vi "灵敏度判定.vi"(0 "曲线引用":refnum<vi>, 1 "灵敏度":T1, 3 "错误输入":errorcluster) -> (7 "曲线引用输出":refnum<vi>, 8 "OK？":bool, 10 "错误输出":errorcluster)   [LabVIEW 2018]
uses:
  Global_Variable/Global.vi
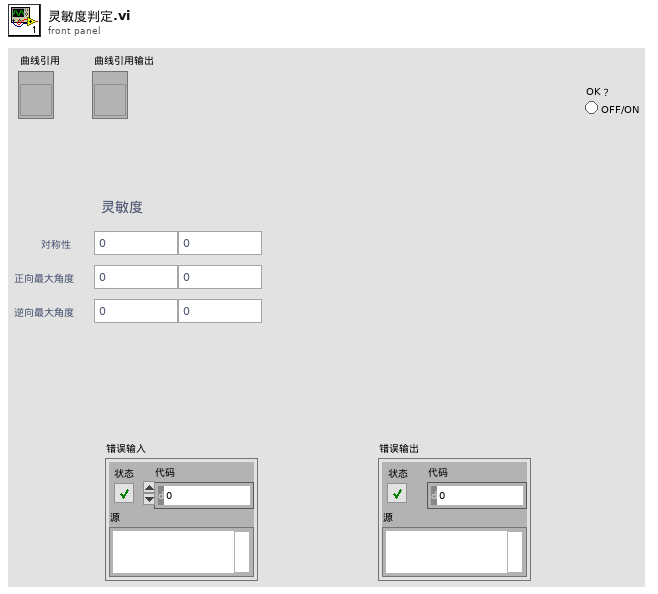
[diagram p1: front panel]
types:
  T1 = cluster{"         对称性":cluster{"下限":dbl, "上限":dbl}, "正向最大角度":cluster{"下限":dbl, "上限":dbl}, "逆向最大角度":cluster{"下限":dbl, "上限":dbl}}
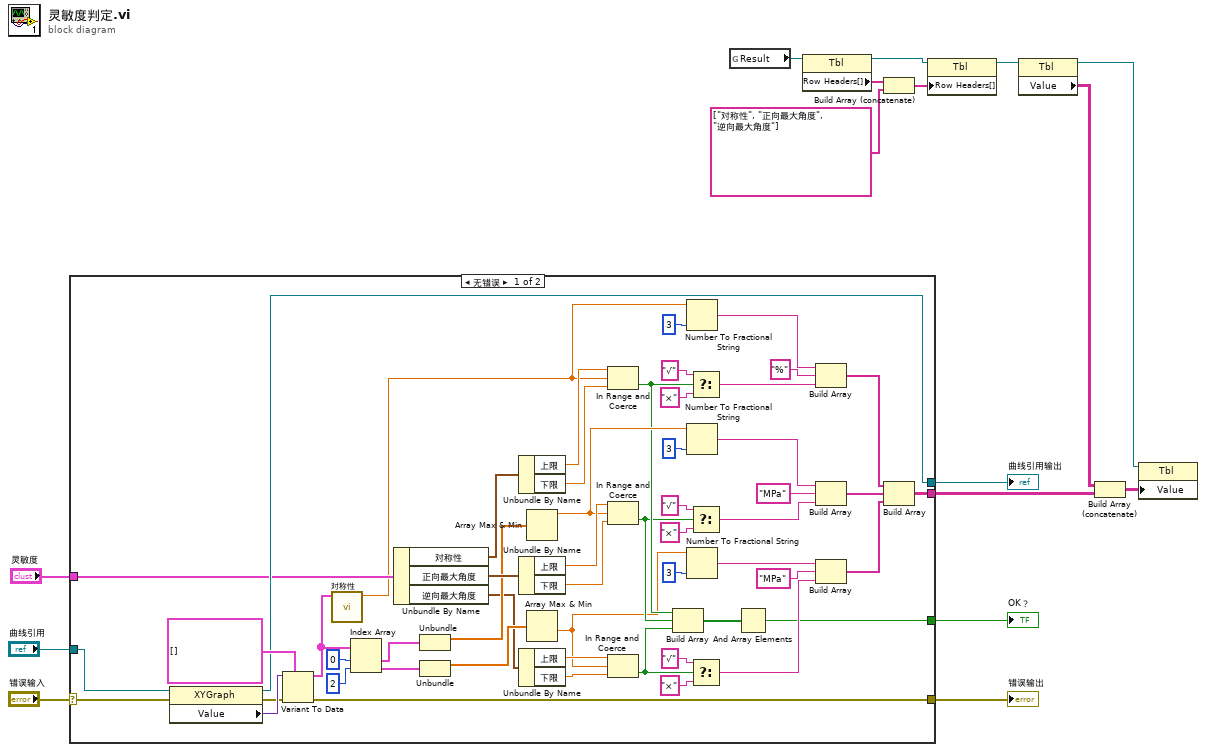
[diagram p0: block diagram]
diagram:
  n1 = case shown="无错误" "错误输入" {
    selector: "错误输入" -> [w68 w72]
    tunnel: [w65 w72] -> w15
    tunnel: "曲线引用" -> [w64 w71]
    tunnel: [w67 w71] -> w13
    tunnel: [w19 _] -> w12
    tunnel: "灵敏度" -> [w63 _]
    tunnel: [w18 _] -> w8
    frame No Error {
      n2 = property class="XYGraph"(reference=w64, error in=w68) -> (reference out=w67:refnum<vi>, error out=w66:errorcluster, "Value"=w70:variant)
      n3 = Variant To Data(error in=w66, type=cluster{dbl[], dbl[]}[] [], Variant=w70) -> (data=w52:cluster{dbl[], dbl[]}[], error out=w65:errorcluster)
      n4 = call "对称性.vi"("XY图"=w52) -> ("对称性"=w59:dbl)  [unwired: 8 in, 2 out]
      n5 = Index Array(array=w52, index #1=0 ("索引"), index #2=2 ("索引")) -> (element #1=w28:cluster{dbl[], dbl[]}, element #2=w27:cluster{dbl[], dbl[]})
      n6 = Unbundle By Name(w63) -> ("对称性"=w62:cluster{"下限":dbl, "上限":dbl}, "正向最大角度"=w43:cluster{"下限":dbl, "上限":dbl}, "逆向最大角度"=w31:cluster{"下限":dbl, "上限":dbl})
      n7 = Unbundle(w28) -> (w42:dbl[])  [unwired: 1 out]
      n8 = Unbundle(w27) -> (w32:dbl[])  [unwired: 1 out]
      n9 = Unbundle By Name(w62) -> ("上限"=w61:dbl, "下限"=w60:dbl)
      n10 = Unbundle By Name(w43) -> ("上限"=w44:dbl, "下限"=w45:dbl)
      n11 = Unbundle By Name(w31) -> ("上限"=w40:dbl, "下限"=w39:dbl)
      n12 = Array Max & Min(array=w42) -> (max value=w41:dbl)  [unwired: 3 out]
      n13 = Array Max & Min(array=w32) -> (min value=w17:dbl)  [unwired: 3 out]
      n14 = In Range and Coerce(upper limit=w61, x=w59, lower limit=w60) -> (In Range?=w25:bool)  [unwired: 1 out]
      n15 = In Range and Coerce(upper limit=w44, x=w41, lower limit=w45) -> (In Range?=w23:bool)  [unwired: 1 out]
      n16 = In Range and Coerce(upper limit=w40, x=w17, lower limit=w39) -> (In Range?=w21:bool)  [unwired: 1 out]
      n17 = Build Array(w25, w23, w21) -> (w20:bool[])
      n18 = Number To Fractional String(number=w59, precision (6)=i16 3 ("精度(6)")) -> (F-format string=w57:string)  [unwired: 2 in]
      n19 = Number To Fractional String(number=w41, precision (6)=i16 3 ("精度(6)")) -> (F-format string=w47:string)  [unwired: 2 in]
      n20 = Number To Fractional String(number=w17, precision (6)=i16 3 ("精度(6)")) -> (F-format string=w37:string)  [unwired: 2 in]
      n21 = Select(t="√" ("元素"), s=w25, f="×" ("元素")) -> (s? t:f=w53:string)
      n22 = Select(t="√" ("元素"), s=w23, f="×" ("元素")) -> (s? t:f=w51:string)
      n23 = Select(t="√" ("元素"), s=w21, f="×" ("元素")) -> (s? t:f=w33:string)
      n24 = And Array Elements(Boolean array=w20) -> (logical AND=w19:bool)
      n25 = Build Array(w57, "%" ("元素"), w53) -> (w26:string[])
      n26 = Build Array(w47, "MPa" ("元素"), w51) -> (w24:string[])
      n27 = Build Array(w37, "MPa" ("元素"), w33) -> (w22:string[])
      n28 = Build Array(w26, w24, w22) -> (w18:string[][])
    }
    frame Error {
    }
  }
  "错误输出" <- w15
  "曲线引用输出" <- w13
  "OK？" <- w12
  n29 = global read "Global.vi" "Result"() -> (w7:refnum<vi>)
  n30 = property class="Tbl"(reference=w7) -> (reference out=w6:refnum<vi>, "Row Headers[]"=w4:string[])  [unwired: 1 in, 1 out]
  n31 = Build Array (concatenate)(w4, string[] ["对称性", "正向最大角度", "逆向最大角度"] ("列首字符串[]")) -> (w2:string[])
  n32 = property class="Tbl"(reference=w6, "Row Headers[]"=w2) -> (reference out=w5:refnum<vi>)  [unwired: 1 in, 1 out]
  n33 = property class="Tbl"(reference=w5) -> (reference out=w11:refnum<vi>, "Value"=w10:string[][])  [unwired: 1 in, 1 out]
  n34 = Build Array (concatenate)(w10, w8) -> (w9:string[][])
  n35 = property class="Tbl"(reference=w11, "Value"=w9) -> ()  [unwired: 1 in, 2 out]
